vi "Bind To Type.vi"(8 "error in (no error)":errorcluster, 10 "Type Name":string, 11 "Flatten To JSON Object in":refnum<class "Flatten To JSON Object.lvclass">) -> (0 "error out":errorcluster, 2 "Type":refnum<class>, 3 "Flatten To JSON Object out":refnum<class "Flatten To JSON Object.lvclass">)   [LabVIEW 2017, in "Flatten To JSON Object.lvclass"]
doc: "Controls the binding of a serialized object to a type."
uses:
  Flatten To JSON Object.lvclass
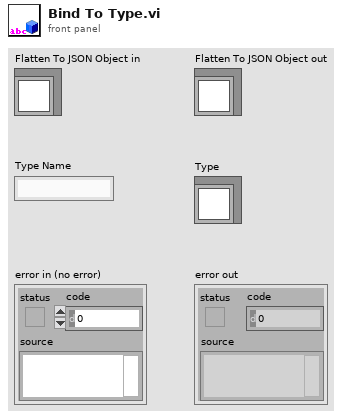
[diagram p1: front panel]
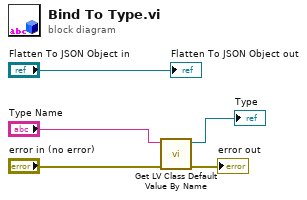
[diagram p0: block diagram]
diagram:
  n1 = call <vilib>:"Get LV Class Default Value By Name.vi"("error in (no error)"="error in (no error)", "class name"="Type Name") -> ("error out"=→"error out":errorcluster, "object"=→"Type":refnum<class>)  [unwired: 8 in]
  "Flatten To JSON Object out" <- "Flatten To JSON Object in"
